vi "subFindProjects.vi"(11 "Path":path) -> (3 "All Files in Dir":path[](array[path]))   [LabVIEW 2020, in "SolutionBuilder.lvlib"]
uses:
  SolutionBuilder.lvlib
  <vilib>/regexp/Match Regular Expression.xnode
  <vilib>/xml/Load XML File.vi
  <vilib>/xml/NI_XML.lvlib
  <vilib>/xml/Close Reference(Node).vi
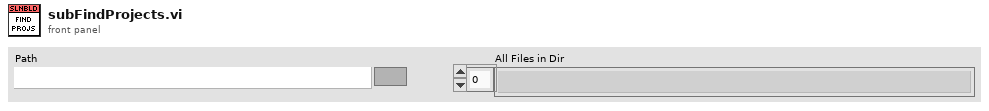
[diagram p1: front panel]
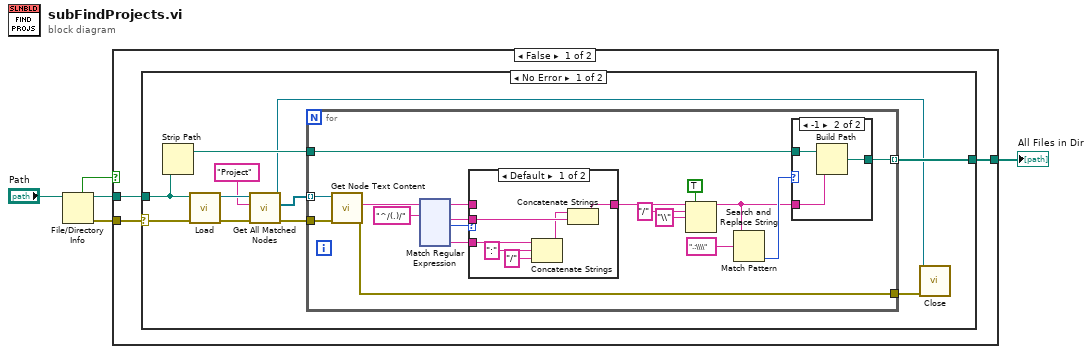
[diagram p0: block diagram]
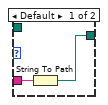
[diagram p3: hidden frame]
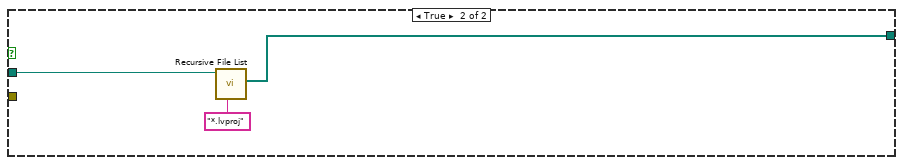
[diagram p5: hidden frame]
diagram:
  n1 = File/Directory Info(path="Path") -> (path out=w2:path, directory=w3:bool, error out=w1:errorcluster)  [unwired: 1 in, 4 out]
  n2 = case shown="False" w3 {
    tunnel: [w6 w167] -> w5
    tunnel: w2 -> [w8 w166]
    tunnel: w1 -> [w7 _]
    frame False {
      n3 = case shown="No Error" w7 {
        selector: w7 -> [w19 _]
        tunnel: w8 -> [w13 _]
        tunnel: [w11 _] -> w6
        frame No Error {
          n4 = Strip Path(path=w13) -> (stripped path=w12:path)  [unwired: 1 out]
          n5 = call-poly <vilib>:"Load.vi"("path to XML document"=w13, "error in (no error)"=w19) -> ("DOM document out"=w18:refnum<k20>, "error out"=w17:errorcluster)  [unwired: 11 in, 1 out]
          n6 = call <vilib>:"Get All Matched Nodes.vi"("error in (no error)"=w17, "XPath expression"="Project", "node in"=w18) -> ("error out"=w15:errorcluster, "node result array"=w14:refnum<k20>[], "node out"=w9:refnum<k20>)  [unwired: 6 in]
          n7 = for {
            tunnel: w15 -> [w37]
            tunnel: w14 -> [w36] mode=indexing
            tunnel: [w32] -> w11 mode=indexing
            tunnel: w12 -> [w33]
            tunnel: [w20] -> w10
            n8 = call <vilib>:"Get Node Text Content.vi"("error in (no error)"=w37, "node in"=w36) -> ("error out"=w20:errorcluster, "node text"=w31:string)  [unwired: 7 in, 1 out]
            n9 = xnode "Match Regular Expression"("input string"=w31, "regular expression"="^/(.)/") -> ("before match"=w28:string, "after match"=w26:string, "offset past match"=w29:i32, "submatch 1"=w27:string)  [unwired: 4 in, 2 out]
            n10 = case shown="Default" w29 {
              tunnel: w28 -> [_ w44]
              tunnel: [w40 w44] -> w25
              tunnel: w27 -> [w42 _]
              tunnel: w26 -> [w43 _]
              frame Default {
                n11 = Concatenate Strings(w42, ":" ("string"), "/" ("string")) -> (w39:string)
                n12 = Concatenate Strings(w39, w43) -> (w40:string)
              }
              frame -1 {
              }
            }
            n13 = Search and Replace String(replace all?=TRUE ("replace all? (F)"), input string=w25, search string="/", replace string="\\" ("replace string (\"\")")) -> (result string=w24:string)  [unwired: 4 in, 3 out]
            n14 = Match Pattern(string=w24, regular expression=".:\\\\") -> (offset past match=w34:i32)  [unwired: 1 in, 3 out]
            n15 = case shown="-1" w34 {
              tunnel: w33 -> [_ w165]
              tunnel: w24 -> [w161 w164]
              tunnel: [w162 w163] -> w32
              frame Default {
                n16 = String To Path(string=w161) -> (path=w162:path)
              }
              frame -1 {
                n17 = Build Path(base path=w165, name or relative path=w164) -> (appended path=w163:path)
              }
            }
          }
          n18 = call-poly <vilib>:"Close.vi"("error in (no error)"=w10, "node"=w9) -> ()  [unwired: 7 in, 1 out]
        }
        frame Error {
        }
      }
    }
    frame True {
      n19 = call <vilib>:"Recursive File List.vi"("pattern"="*.lvproj", "Folder Path"=w166) -> ("All Files in Dir"=w167:path[])  [unwired: 5 in, 4 out]
    }
  }
  "All Files in Dir" <- w5
